vi "02 - Getting an image on the screen.vi"() -> ()   [LabVIEW 2015]
uses:
  Libraries/LibSDL2 Wrapper/Controls/Init Flags.ctl
  Libraries/LibSDL2 Wrapper/Controls/NULL.ctl
  Libraries/LibSDL2 Wrapper/LibSDL2.lvlib
panel:
  out "Error":string
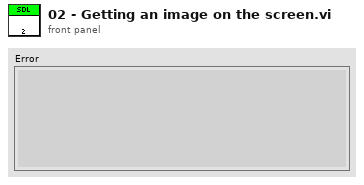
[diagram p1: front panel]
types:
  T1 = typedef "LibSDL2.lvlib/NULL.ctl" = enum32{"NULL"}
  T2 = typedef "LibSDL2.lvlib/Init Flags.ctl" = u32
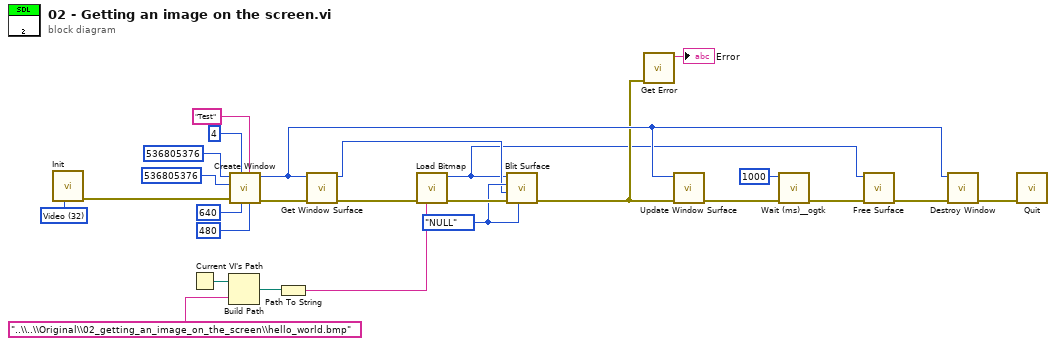
[diagram p0: block diagram]
diagram:
  w9 = NULL."NULL" ("Null")
  w26 = T2 32 items=["Timer"=1, "Audio"=16, "Video"=32, "Joystick"=512, "Haptic"=4096, "Game Controller"=8192, "Events"=16384, "No Parachute"=1048576, "Everything"=17244689] ("Init Flags")
  n1 = call "Init.vi"("Flags"=w26) -> ("error out"=w20:errorcluster)  [unwired: 9 in, 1 out]
  n2 = Current VI's Path() -> (path=w4:path)
  n3 = Build Path(base path=w4, name or relative path="..\\..\\Original\\02_getting_an_image_on_the_screen\\hello_world.bmp" ("File")) -> (appended path=w2:path)
  n4 = call "Create Window.vi"("Height"=480, "Title"="Test", "Width"=640, "Flags"=u32 4, "error in"=w20, "Position y"=u32 536805376 ("Flags"), "Position x"=u32 536805376 ("Flags")) -> ("error out"=w13:errorcluster, "Window Pointer"=w15:u32)  [unwired: 3 in]
  n5 = Path To String(path=w2) -> (string=w1:string)
  n6 = call "Get Window Surface.vi"("error in"=w13, "Window Pointer"=w15) -> ("error out"=w12:errorcluster, "Surface Pointer"=w6:u32)  [unwired: 8 in]
  n7 = call "Load Bitmap.vi"("error in"=w12, "File"=w1) -> ("error out"=w11:errorcluster, "Surface Pointer"=w5:u32)  [unwired: 8 in]
  n8 = call "Blit Surface.vi"("Destination Rectangle Pointer"=w9, "error in"=w11, "Destination Surface Pointer"=w6, "Source Rectangle Pointer"=w9, "Source Surface Pointer"=w5) -> ("error out"=w10:errorcluster)  [unwired: 5 in, 1 out]
  n9 = call "Get Error.vi"("error in"=w10) -> ("Error"=→"Error":string)  [unwired: 9 in, 1 out]
  n10 = call "Update Window Surface.vi"("error in"=w10, "Window Pointer"=w15) -> ("error out"=w17:errorcluster)  [unwired: 9 in]
  n11 = call <userlib>:"Wait (ms)__ogtk.vi"("error in (no error)"=w17, "milliseconds to wait"=u32 1000) -> ("error out"=w8:errorcluster)  [unwired: 8 in, 1 out]
  n12 = call "Free Surface.vi"("error in"=w8, "Surface Pointer"=w5) -> ("error out"=w7:errorcluster)  [unwired: 9 in]
  n13 = call "Destroy Window.vi"("error in"=w7, "Window Pointer"=w15) -> ("error out"=w16:errorcluster)  [unwired: 9 in]
  n14 = call "Quit.vi"("error in"=w16) -> ()  [unwired: 10 in, 1 out]
